vi "Compare LabVIEW File.vi"(6 "Interactive?":bool, 7 "Export Images?":bool, 8 "error in":errorcluster, 10 "Results Directory":path, 11 "File Info in":T1) -> (0 "error out":errorcluster, 3 "File Info out":T1)   [LabVIEW 2020, in "Peer Review.lvclass"]
uses:
  Peer Review.lvclass
  TypeDefs/File Info.ctl
  TypeDefs/File State.ctl
  TypeDefs/VI Type.ctl
  <vilib>/Utility/error.llb/Trim Whitespace One-Sided.vi
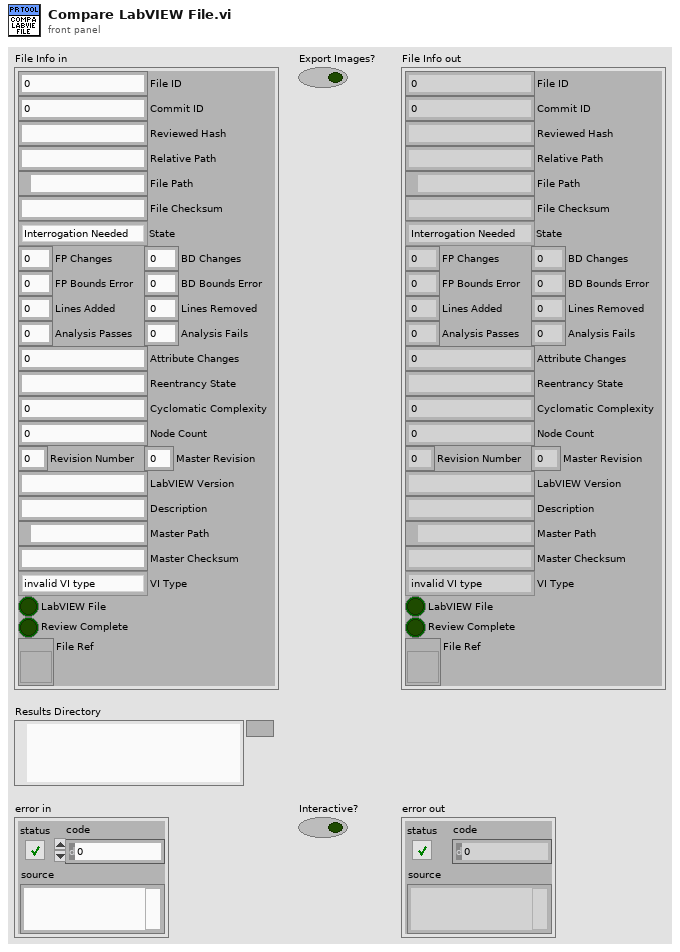
[diagram p1: front panel]
types:
  T1 = typedef "Peer Review.lvclass/File Info.ctl" = cluster{"File ID":i32, "Commit ID":i32, "Reviewed Hash":string, "Relative Path":string, "File Path":path, "File Checksum":string, "State":T2, "FP Changes":i32, "BD Changes":i32, "FP Bounds Error":dbl, "BD Bounds Error":dbl, "Lines Added":i32, "Lines Removed":i32, "Analysis Passes":i32, "Analysis Fails":i32, "Attribute Changes":i32, "Reentrancy State":string, "Cyclomatic Complexity":i32, "Node Count":i32, "Revision Number":u32, "LabVIEW Version":string, "Description":string, "Master Path":path, "Master Checksum":string, "VI Type":T3, "LabVIEW File":bool, "Review Complete":bool, "File Ref":refnum<vi>, "Master Revision":u32}
  T2 = typedef "Peer Review.lvclass/File State.ctl" = enum16{"Interrogation Needed", "Modified", "Deleted", "Added", "Matches Previous", "No Changes", "Moved", "Empty File"}
  T3 = typedef "Peer Review.lvclass/VI Type.ctl" = enum32{"invalid VI type", "Standard VI", "Control VI", "Global VI", "Polymorphic VI", "Configuration VI", "SubSystem", "Facade VI", "Method VI", "Statechart Diagram VI"}
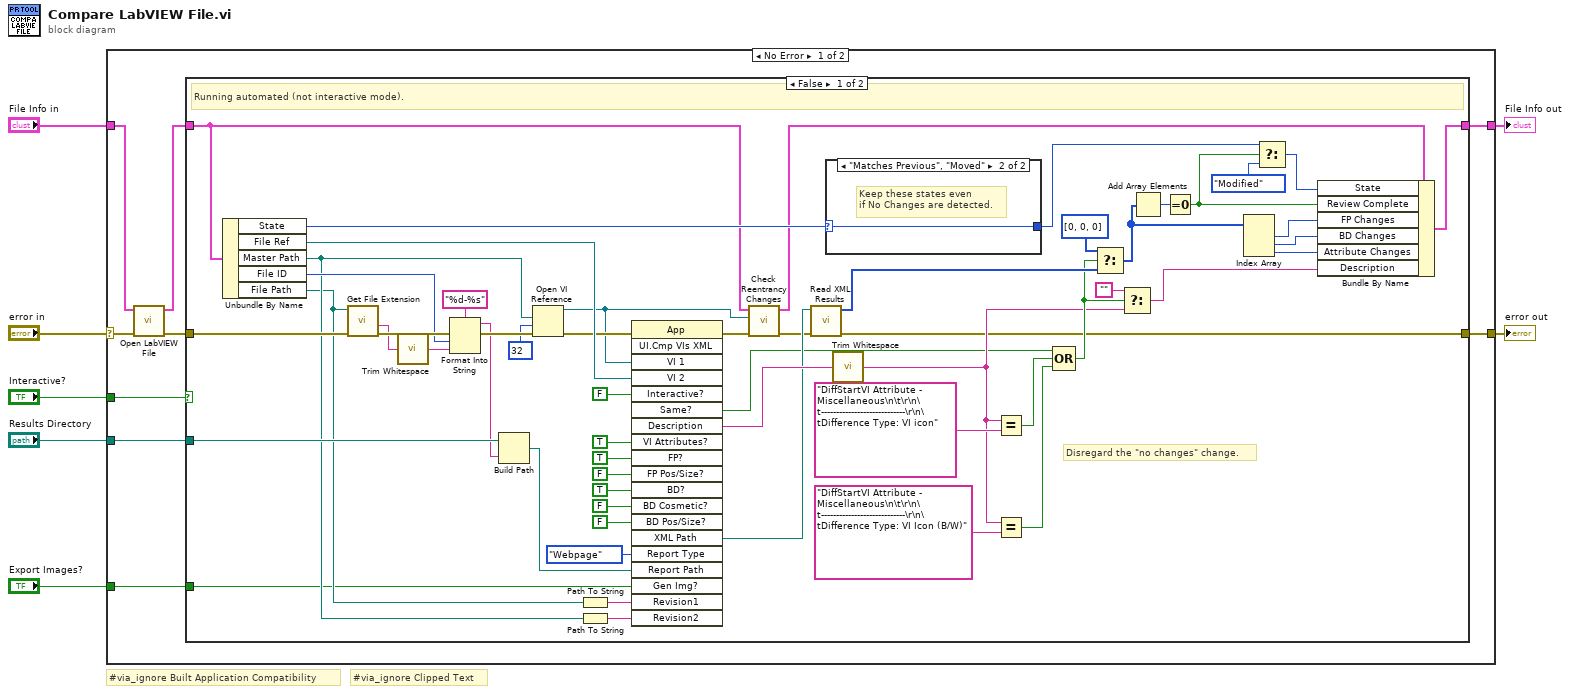
[diagram p0: block diagram]
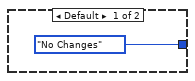
[diagram p2: hidden frame]
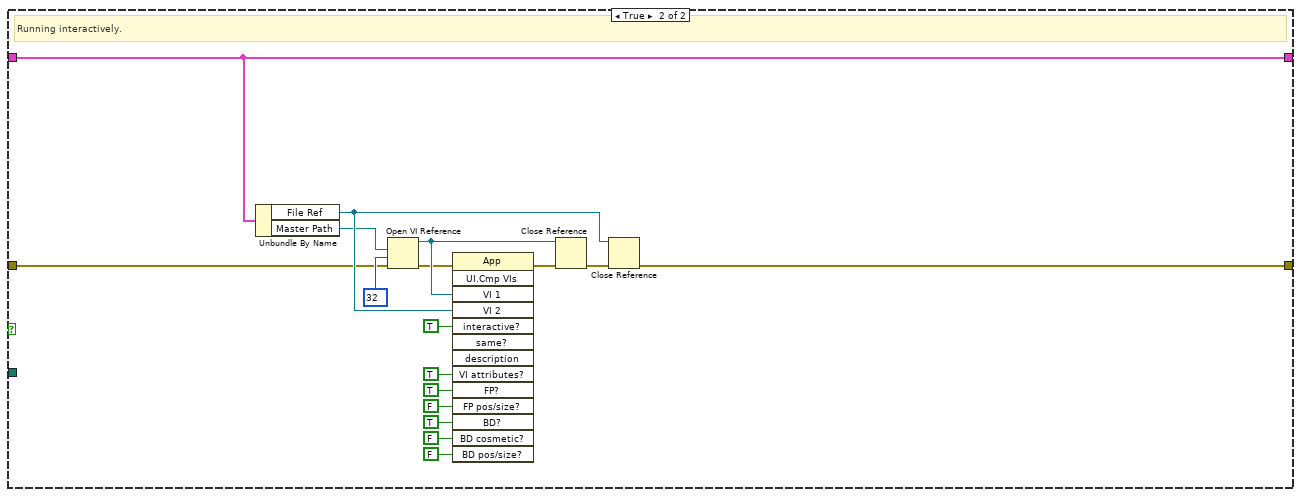
[diagram p3: hidden frame]
diagram:
  # "#via_ignore Clipped Text"
  # "#via_ignore Built Application Compatibility"
  n1 = case shown="No Error" "error in" {
    selector: "error in" -> [w12 w93]
    tunnel: "File Info in" -> [w9 w92]
    tunnel: "Interactive?" -> [w13 _]
    tunnel: [w16 w92] -> w5
    tunnel: [w15 w93] -> w4
    tunnel: "Results Directory" -> [w14 _]
    tunnel: "Export Images?" -> [w8 _]
    frame No Error {
      n2 = call "Open LabVIEW File.vi"("error in"=w12, "File Info in"=w9) -> ("error out"=w11:errorcluster, "File Info out"=w10:T1)  [unwired: 8 in]
      n3 = case shown="False" w13 {
        tunnel: [w24 w78] -> w16
        tunnel: [w25 w80] -> w15
        tunnel: w14 -> [w70 _]
        tunnel: w11 -> [w67 w76]
        tunnel: w10 -> [w22 w78]
        tunnel: w8 -> [w17 _]
        frame False {
          # "Disregard the \"no changes\" change."
          # "Running automated (not interactive mode)."
          n4 = Unbundle By Name(w22) -> ("State"=w56:T2, "File Ref"=w48:refnum<vi>, "Master Path"=w51:path, "File ID"=w55:i32, "File Path"=w18:path)
          n5 = call <vilib>:"Get File Extension.vi"("error in (no error)"=w67, "file"=w18) -> ("error out"=w68:errorcluster, "filename without extension"=w54:string)  [unwired: 5 in, 3 out]
          n6 = call <vilib>:"Trim Whitespace.vi"("string"=w54) -> ("trimmed string"=w53:string)  [unwired: 1 in]
          n7 = Format Into String(format string="%d-%s", error in=w68, w55, w53) -> (resulting string=w52:string, error out=w66:errorcluster)  [unwired: 1 in]
          n8 = Build Path(base path=w70, name or relative path=w52) -> (appended path=w69:path)
          n9 = Open VI Reference(vi path=w51, options=32, error in (no error)=w66) -> (vi reference=w21:refnum<vi>, error out=w47:errorcluster)  [unwired: 1 in, 2 out]
          n10 = Path To String(path=w18) -> (string=w64:string)
          n11 = Path To String(path=w51) -> (string=w65:string)
          n12 = invoke on="Invoke Node" class="App" method="UI.Cmp VIs XML"(error in=w47, "VI 1"=w21, "VI 2"=w48, "Interactive?"=FALSE, "VI Attributes?"=TRUE, "FP?"=TRUE, "FP Pos/Size?"=FALSE, "BD?"=TRUE, "BD Cosmetic?"=FALSE, "BD Pos/Size?"=FALSE, "Report Type"=enum32{"None", "Webpage", "Text", "MS Word"}."Webpage", "Report Path"=w69, "Gen Img?"=w17, "Revision1"=w64, "Revision2"=w65) -> (error out=w49:errorcluster, "Same?"=w19:bool, "Description"=w72:string, "XML Path"=w50:path)  [unwired: 5 in, 16 out]
          n13 = call "Check Reentrancy Changes.vi"("error in"=w49, "Master VI Ref"=w21, "File Info in"=w22) -> ("error out"=w27:errorcluster, "File Info out"=w23:T1)  [unwired: 7 in]
          n14 = call "Read XML Results.vi"("error in"=w27, "XML Path"=w50) -> ("error out"=w25:errorcluster, "Changes"=w32:i32[])  [unwired: 8 in]
          n15 = case shown="\"Matches Previous\", \"Moved\"" w56 {
            selector: w56 -> [_ w74]
            tunnel: [File_State."No Changes" ("f") w74] -> w26
            frame Default {
            }
            frame "Matches Previous", "Moved" {
              # "Keep these states even\nif No Changes are detected."
            }
          }
          n16 = call <vilib>:"Trim Whitespace.vi"("string"=w72) -> ("trimmed string"=w28:string)  [unwired: 1 in]
          n17 = Equal?(x=w28, y="DiffStartVI Attribute - Miscellaneous\n\t\r\n\t----------------------------\r\n\tDifference Type: VI icon" ("Display")) -> (x = y?=w37:bool)
          n18 = Equal?(x=w28, y="DiffStartVI Attribute - Miscellaneous\n\t\r\n\t----------------------------\r\n\tDifference Type: VI Icon (B/W)" ("Description")) -> (x = y?=w38:bool)
          n19 = Compound Arithmetic op=OR(w19, w37, w38) -> (w29:bool)
          n20 = Select(t=i32[] [0, 0, 0] ("Changes"), s=w29, f=w32) -> (s? t:f=w30:i32[])
          n21 = Select(t="" ("Empty String Constant"), s=w29, f=w28) -> (s? t:f=w31:string)
          n22 = Add Array Elements(numeric array=w30) -> (sum=w44:i32)
          n23 = Equal To 0?(x=w44) -> (x = 0?=w35:bool)
          n24 = Index Array(array=w30) -> (element #1=w41:i32, element #2=w42:i32, element #3=w43:i32)  [unwired: 3 in]
          n25 = Select(t=w26, s=w35, f=File_State."Modified") -> (s? t:f=w36:T2)
          n26 = Bundle By Name(cluster=w23, "State"=w36, "Review Complete"=w35, "FP Changes"=w41, "BD Changes"=w42, "Attribute Changes"=w43, "Description"=w31) -> (w24:T1)
        }
        frame True {
          # "Running interactively."
          n27 = Unbundle By Name(w78) -> ("File Ref"=w77:refnum<vi>, "Master Path"=w75:path)
          n28 = Open VI Reference(vi path=w75, options=32, error in (no error)=w76) -> (vi reference=w84:refnum<vi>, error out=w82:errorcluster)  [unwired: 1 in, 2 out]
          n29 = invoke on="Invoke Node" class="App" method="UI.Cmp VIs"(error in=w82, "VI 1"=w84, "VI 2"=w77, "interactive?"=TRUE ("Interactive?"), "VI attributes?"=TRUE ("VI Attributes?"), "FP?"=TRUE, "FP pos/size?"=FALSE ("FP Pos/Size?"), "BD?"=TRUE, "BD cosmetic?"=FALSE ("BD Cosmetic?"), "BD pos/size?"=FALSE ("BD Pos/Size?")) -> (error out=w85:errorcluster)  [unwired: 4 in, 13 out]
          n30 = Close Reference(reference=w84, error in (no error)=w85) -> (error out=w81:errorcluster)
          n31 = Close Reference(reference=w77, error in (no error)=w81) -> (error out=w80:errorcluster)
        }
      }
    }
    frame Error {
    }
  }
  "File Info out" <- w5
  "error out" <- w4
